vi "Init Client.vi"(5 "EventLogger":refnum<class "EventLoggingService.lvclass">, 7 "SequenceCountService":refnum<class "SequenceCountService.lvclass">, 8 "error in (no error)":errorcluster, 9 "Remote Port":u16, 10 "Remote Address":string, 11 "Client Info":T1) -> (0 "error out":errorcluster, 3 "TCPMessaging out":refnum<class "TCPMessaging.lvclass">)   [LabVIEW 2020, in "Vecto.lvlib" / "TCPMessaging.lvclass"]
uses:
  TCPMessaging.lvclass
  proto/TcpClientHello/Data.ctl
  SequenceCountService/SequenceCountService.lvclass
  EventLoggingService/EventLoggingService.lvclass
  TCP Mode.ctl
  Event Level.ctl
  TCPMessaging.lvclass/TCPMessaging.ctl
  EventLoggingService/EventLoggingService.lvclass/EventLoggingService.ctl
  <vilib>/Utility/error.llb/Error Cluster From Error Code.vi
  EventLogHandler/EventLogHandler.lvclass
  Vecto.lvlib
  proto/TcpClientHello/TcpClientHello.lvlib
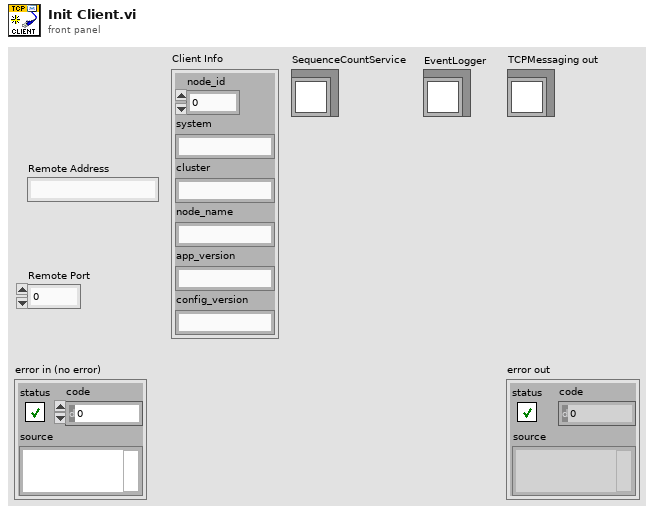
[diagram p1: front panel]
types:
  T1 = typedef "TcpClientHello.lvlib/Data.ctl" = cluster{"node_id":u32, "system":string, "cluster":string, "node_name":string, "app_version":string, "config_version":string}
  T2 = typedef "Vecto.lvlib/Event Level.ctl" = enum16{"Debug", "Info", "Warning", "Error"}
  T3 = typedef "Vecto.lvlib/TCPMessaging.lvclass/TCP Mode.ctl" = enum16{"Client", "Server"}
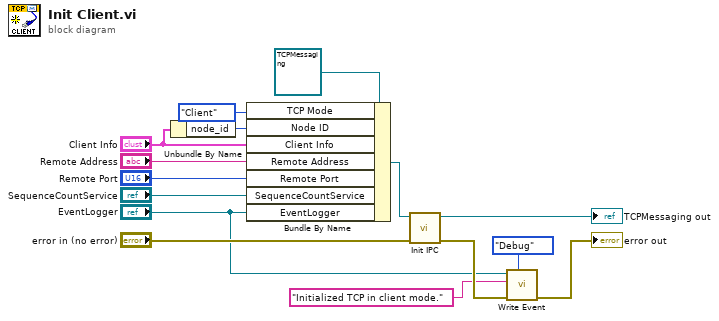
[diagram p0: block diagram]
diagram:
  n1 = Unbundle By Name("Client Info") -> ("node_id"=w6:u32)
  n2 = Bundle By Name(cluster=refnum<class "TCPMessaging.lvclass"> refnum ("TCPMessaging in"), "TCP Mode"=TCP_Mode."Client", "Node ID"=w6, "Client Info"="Client Info", "Remote Address"="Remote Address", "Remote Port"="Remote Port", "SequenceCountService"="SequenceCountService", "EventLogger"="EventLogger") -> (w9:refnum<class "TCPMessaging.lvclass">)
  n3 = call "Init IPC.vi"("error in (no error)"="error in (no error)", "TCPMessaging in"=w9) -> ("error out"=w10:errorcluster, "TCPMessaging out"=→"TCPMessaging out":refnum<class "TCPMessaging.lvclass">)  [unwired: 8 in]
  n4 = call "Write Event.vi"("Event Level (Info)"=Event_Level."Debug", "error in (no error)"=w10, "Message"="Initialized TCP in client mode.", "EventLoggingService in"="EventLogger") -> ("error out"=→"error out":errorcluster)  [unwired: 6 in, 1 out]
